vi "calculate AO1 laser waveform.vi"(8 "error in (no error)":errorcluster, 11 "NI in":refnum<class "NI.lvclass">) -> (0 "error out":errorcluster, 3 "NI out":refnum<class "NI.lvclass">)   [LabVIEW 2021, in "NI.lvlib" / "NI.lvclass"]
uses:
  NI.lvclass
  NI.lvclass/NI.ctl
panel:
  out "waveform":i16[][](graph)
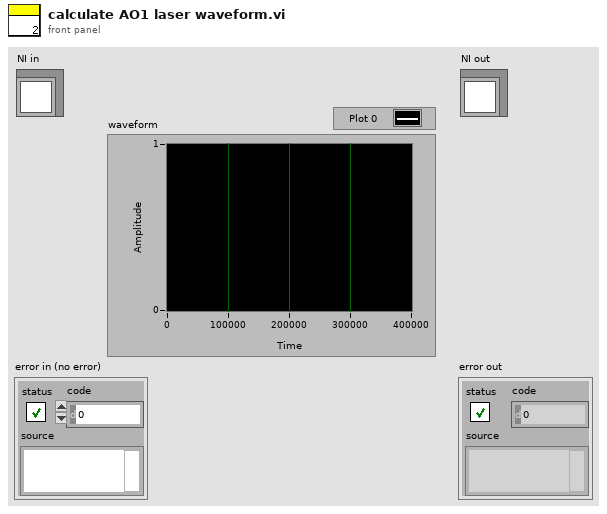
[diagram p1: front panel]
types:
  T1 = typedef "NI.lvlib/NI.lvclass/NI task parameters.ctl" = cluster{"exposure time":dbl, "camera H":dbl, "y line #":dbl, "flyback line #":dbl, "y pixel size":dbl, "z scan #":dbl, "z step size":dbl, "z offset":dbl, "laser all on?":bool, "laser option":bool[]}
  T2 = typedef "NI.lvlib/NI.lvclass/Channel Connection.ctl" = cluster{"Physical Channel":tag, "Terminal":tag, "StartTrigger":tag, "ClockSource":tag}
  T3 = cluster{"fast clock params":cluster{"fast clock rate":dbl, "off time after trigger":dbl, "cam line read time":dbl, "protect ticks #":dbl}, "AO1 laser Connection":T2, "AO2 zy Connection":T2, "AO3 z Connection (deprecated)":T2, "CO1 mainTrig Connection":T2, "CO2 fastClock Connection":T2, "AI phase Connection":T2}
  T4 = cluster{"fast clock rate":dbl, "off time after trigger":dbl, "cam line read time":dbl, "protect ticks #":dbl}
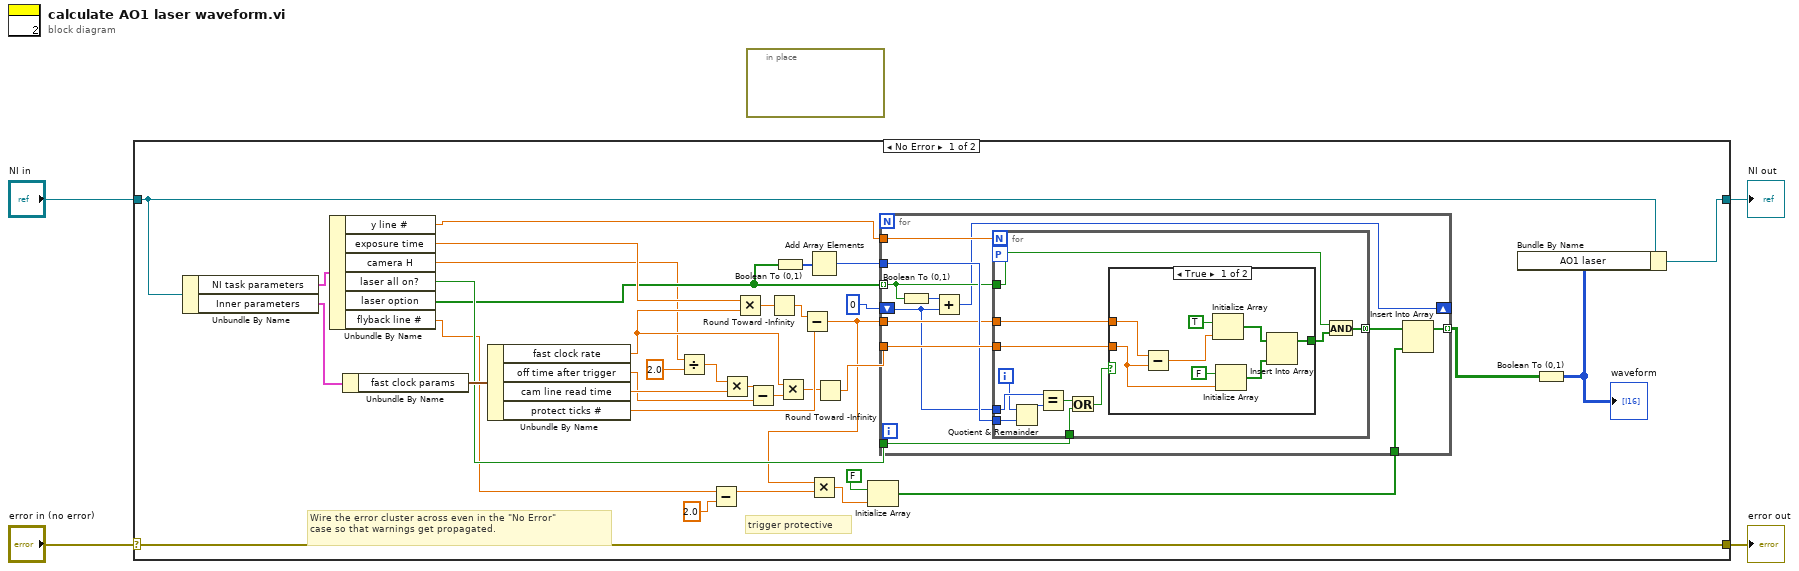
[diagram p0: block diagram]
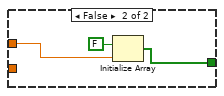
[diagram p2: hidden frame]
diagram:
  n1 = case shown="No Error" "error in (no error)" {
    selector: "error in (no error)" -> [w39 w76]
    tunnel: [w39 w76] -> w3
    tunnel: [w21 w75] -> w1
    tunnel: "NI in" -> [w22 w75]
    frame No Error {
      # "trigger protective"
      # "Wire the error cluster across even in the \"No Error\"\ncase so that warnings get propagated."
      n2 = Unbundle By Name(w22) -> ("NI task parameters"=w38:T1, "Inner parameters"=w37:T3)
      n3 = Unbundle By Name(w38) -> ("y line #"=w26:dbl, "exposure time"=w35:dbl, "camera H"=w9:dbl, "laser all on?"=w23:bool, "laser option"=w15:bool[], "flyback line #"=w18:dbl)
      n4 = Unbundle By Name(w37) -> ("fast clock params"=w34:T4)
      n5 = Unbundle By Name(w34) -> ("fast clock rate"=w27:dbl, "off time after trigger"=w29:dbl, "cam line read time"=w31:dbl, "protect ticks #"=w32:dbl)
      n6 = Divide(x=w9, y=2.0) -> (x/y=w8:dbl)
      n7 = Subtract(x=w18, y=2.0) -> (x-y=w6:dbl)
      n8 = Multiply(x=w8, y=w31) -> (x*y=w30:dbl)
      n9 = Multiply(x=w35, y=w27) -> (x*y=w36:dbl)
      n10 = Subtract(x=w30, y=w29) -> (x-y=w28:dbl)
      n11 = Round Toward -Infinity(1:w36) -> (0:w33:dbl)
      n12 = Boolean To (0,1)(Boolean=w15) -> (0, 1=w14:i16[])
      n13 = Multiply(x=w27, y=w28) -> (x*y=w25:dbl)
      n14 = Subtract(x=w33, y=w32) -> (x-y=w16:dbl)
      n15 = Add Array Elements(numeric array=w14) -> (sum=w13:i16)
      n16 = Multiply(x=w16, y=w6) -> (x*y=w17:dbl)
      n17 = Round Toward -Infinity(1:w25) -> (0:w24:dbl)
      n18 = Initialize Array(FALSE ("element"), w17) -> (w10:bool[])
      n19 = for {
        tunnel: w15 -> [w46] mode=indexing
        tunnel: w24 -> [w51]
        tunnel: w16 -> [w47]
        tunnel: w23 -> [w50]
        tunnel: [w42] -> w11 mode=indexing
        tunnel: w26 -> [w49]
        tunnel: w13 -> [w48]
        shift-right: [w44] -> _
        shift-left: i16 0 ("0, 1") -> [w43]
        tunnel: w10 -> [w40]
        n20 = Boolean To (0,1)(Boolean=w46) -> (0, 1=w45:i16)
        n21 = Add(x=w45, y=w43) -> (x+y=w44:i16)
        n22 = for {
          N: w49 -> [_]
          tunnel: w46 -> [w56]
          tunnel: w51 -> [w62]
          tunnel: w47 -> [w63]
          tunnel: w43 -> [w54]
          tunnel: w50 -> [w59]
          tunnel: [w55] -> w41 mode=concatenating
          tunnel: w48 -> [w52]
          workers-P: _ -> [_]
          i -> [w53]
          n23 = Quotient & Remainder(x=w53, y=w52) -> (x-y*floor(x/y)=w61:i32)  [unwired: 1 out]
          n24 = Equal?(x=w54, y=w61) -> (x = y?=w60:bool)
          n25 = Or(x=w60, y=w59) -> (x .or. y?=w58:bool)
          n26 = case shown="True" w58 {
            tunnel: w63 -> [w67 w73]
            tunnel: w62 -> [w65 _]
            tunnel: [w66 w72] -> w57
            frame True {
              n27 = Subtract(x=w67, y=w65) -> (x-y=w64:dbl)
              n28 = Initialize Array(TRUE ("element"), w64) -> (w71:bool[])
              n29 = Initialize Array(FALSE ("element"), w65) -> (w70:bool[])
              n30 = Insert Into Array(array=w71, new element=w70) -> (w66:bool[])  [unwired: 1 in]
            }
            frame False {
              n31 = Initialize Array(FALSE ("element"), w73) -> (w72:bool[])
            }
          }
          n32 = And(x=w56, y=w57) -> (x .and. y?=w55:bool[])
        }
        n33 = Insert Into Array(array=w41, new element=w40) -> (w42:bool[])  [unwired: 1 in]
      }
      n34 = Boolean To (0,1)(Boolean=w11) -> (0, 1=w19:i16[][])
      "waveform" <- w19
      n35 = Bundle By Name(cluster=w22, "AO1 laser"=w19) -> (w21:refnum<class "NI.lvclass">)
    }
    frame Error {
    }
  }
  "error out" <- w3
  "NI out" <- w1
  n36 = in-place {
  }
